vi "Draw ROI.vi"(8 "Error In":errorcluster, 9 "Right Border location (pix)":i32, 10 "Horizontal Line location (pix)":i32) -> (0 "Error Out":errorcluster, 2 "ROI Descriptor":T1 {"Contours"."Type" items=["No Selection", "Point", "Line", "Rectangle", "Oval", "Polygon", "Freehand Region", "Annulus", "Unused2", "Unused3", "Broken Line", "Freehand Line", "Rotated Rectangle"]}, 3 "Image Out":T2(plugin-control))   [LabVIEW 2018, in "Image Management.lvlib"]
uses:
  Image Management.lvlib
  Action.ctl
  ROI Info--cluster.ctl
  <vilib>/vision/Image Controls.llb/IMAQ Image.ctl
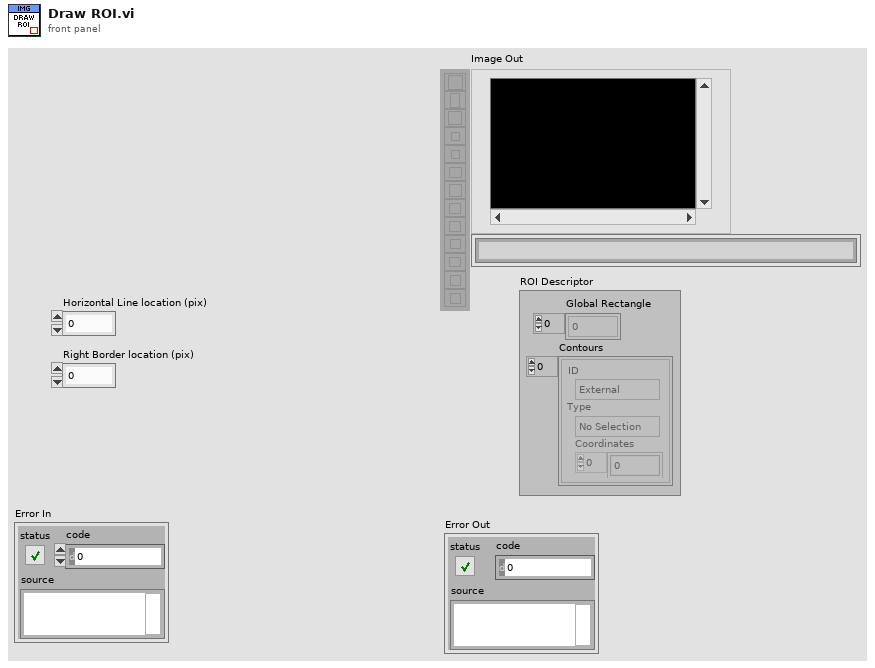
[diagram p1: front panel]
types:
  T1 = typedef "ROI Descriptor" = cluster{"Global Rectangle":i32[], "Contours":cluster{"ID":enum32{"External", "Internal"}, "Type":u32, "Coordinates":i32[]}[]}
  T2 = typedef "IMAQ Image.ctl" = refnum<image>
  T3 = typedef "Image Management.lvlib/ROI Info--cluster.ctl" = cluster{"Horizontal Line Location (pix)":i32, "Right Border Location (pix)":i32}
  T4 = typedef "Image Management.lvlib/Action.ctl" = enum16{"Init", "Output Image Path", "Open Image in Default Program", "Find Linespaces", "Get Image Size (pixels)", "Draw ROIs", "Make Section Images", "Close"}
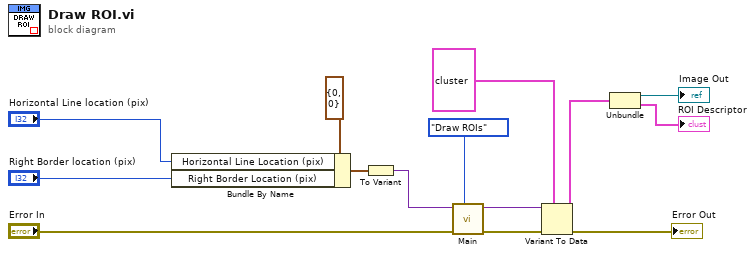
[diagram p0: block diagram]
diagram:
  n1 = Bundle By Name(cluster=T3 {"Horizontal Line Location (pix)"=0, "Right Border Location (pix)"=0} ("ROI info"), "Horizontal Line Location (pix)"="Horizontal Line location (pix)", "Right Border Location (pix)"="Right Border location (pix)") -> (w5:T3)
  n2 = To Variant(anything=w5) -> (Variant=w9:variant)
  n3 = call "Main.vi"("Action"=Action."Draw ROIs", "Error In"="Error In", "Data in"=w9) -> ("Error Out"=w13:errorcluster, "Output"=w12:variant)  [unwired: 7 in]
  n4 = Variant To Data(error in=w13, type=cluster{"Refnum out":T2, "ROI Descriptor":T1} {"Refnum out"=refnum, "ROI Descriptor"={"Global Rectangle"=[], "Contours"=[]}} ("cluster"), Variant=w12) -> (data=w3:cluster{"Refnum out":T2, "ROI Descriptor":T1}, error out=→"Error Out":errorcluster)
  n5 = Unbundle(w3) -> ("Refnum out"=→"Image Out":T2, "ROI Descriptor"=→"ROI Descriptor":T1)
